vi "LVClass_DataClient GetSlopes.vi"(0 "DataClient in":refnum<class "DataClient.lvclass">, 5 "name":string, 7 "HasoSlopes in":refnum<class "HasoSlopes.lvclass">, 11 "error in (no error)":errorcluster) -> (4 "DataClient out":refnum<class "DataClient.lvclass">, 8 "HasoSlopes (dup)":refnum<class "HasoSlopes.lvclass">, 10 "data_unique_id":i32, 15 "error out":errorcluster)   [LabVIEW 2020, in "DataClient.lvclass"]
doc: "Slopes getter.\n\n--------------------------------------------------------------------------------\n\n<B>clientIn </B> : Client object.\n<B>clientOut </B> : Client object.\n<B>hasoslopes </B> : HasoSlopes object.\n<B>ErrorIn </B> : Error\n<B>ErrorOut </B> : Error\n\n--------------------------------------------------------------------------------"
uses:
  DataClient.lvclass
  HasoSlopes.lvclass
  DataClient.lvclass/DataClient.ctl
  LVClass_HasoSlopes Read HasoSlopes _ property.vi
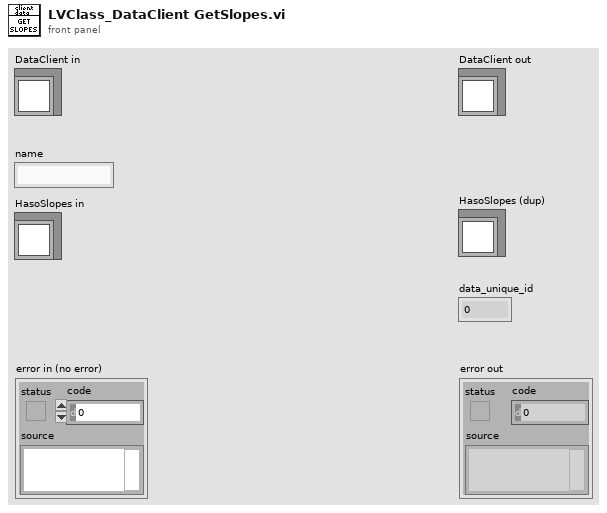
[diagram p1: front panel]
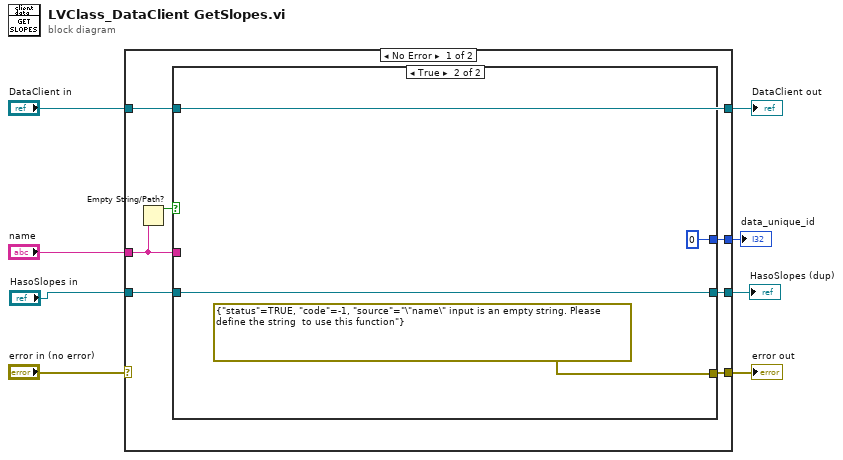
[diagram p0: block diagram]
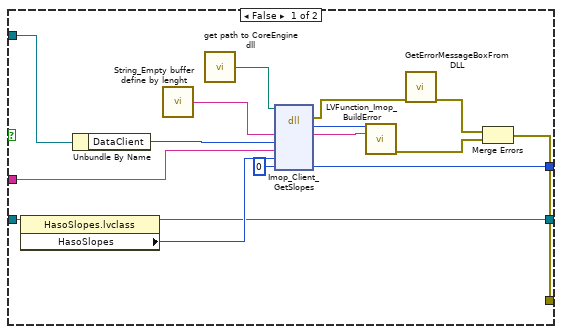
[diagram p2: hidden frame]
diagram:
  n1 = case shown="No Error" "error in (no error)" {
    selector: "error in (no error)" -> [_ w37]
    tunnel: [w13 w37] -> w7
    tunnel: [w15 w36] -> w5
    tunnel: "DataClient in" -> [w15 w36]
    tunnel: "HasoSlopes in" -> [w14 w35]
    tunnel: [w11 w35] -> w3
    tunnel: "name" -> [w10 _]
    tunnel: [w12 _] -> w1
    frame No Error {
      n2 = Empty String/Path?(string/path=w10) -> (empty?=w9:bool)
      n3 = case shown="True" w9 {
        tunnel: w15 -> [w22 _]
        tunnel: w14 -> [w21 w34]
        tunnel: [w20 errorcluster {"status"=TRUE, "code"=-1, "source"="\"name\" input is an empty string. Please define the string  to use this function"} ("error IO")] -> w13
        tunnel: [w18 0 ("data_id")] -> w12
        tunnel: [w17 w34] -> w11
        tunnel: w10 -> [w16 _]
        frame False {
          n4 = property class="HasoSlopes.lvclass"(reference=w21) -> (reference out=w17:refnum<class "HasoSlopes.lvclass">, "HasoSlopes"=w31:i32)  [unwired: 1 in, 1 out]
          n5 = Unbundle By Name(w22) -> ("DataClient"=w25:i32)
          n6 = call "String_Empty buffer define by lenght.vi"() -> ("Empty buffer"=w28:string)  [unwired: 1 in]
          n7 = call "get path to CoreEngine dll.vi"() -> ("path to c_interface_vc100.dll"=w27:path)  [unwired: 12 in, 3 out]
          n8 = dll-call lib="D:/soft/HASO_v3/SVN_trunk/ImOpCoreEngine4_LV2011/DLLs/c_interface_vc100.dll" fn="Imop_Client_GetSlopes"(path in=w27, "message"=w28, "client"=w25, "name"=w16, "HasoSlopes"=w31, "data_id"=0) -> (error out=w26:errorcluster, "return type"=w30:i32, "message"=w29:string, "data_id"=w18:i32)  [unwired: 5 in, 1 out]
          n9 = call "LVFunction_Imop_BuildError.vi"("code"=w30, "String to Prepend to source (\"\")"=w29) -> ("error out"=w23:errorcluster)  [unwired: 13 in]
          n10 = call "GetErrorMessageBoxFromDLL.vi"("error IN"=w26) -> ("error OUT"=w24:errorcluster)  [unwired: 10 in]
          n11 = Merge Errors(w24, w23) -> (w20:errorcluster)
        }
        frame True {
        }
      }
    }
    frame Error {
    }
  }
  "error out" <- w7
  "DataClient out" <- w5
  "HasoSlopes (dup)" <- w3
  "data_unique_id" <- w1
